vi "LIA_Initialization.vi"(8 "error in (no error)":errorcluster, 10 "Lock-in Parameters":T3[](array[typedef]) {"Value" format="%#_6p"}, 11 "Address":string) -> (0 "error out":errorcluster, 1 "Selected Device":string, 2 "DAQ ModHandle Out":T1 {"ModHandle" format="0x%08x"; "Conn" format="0x%08x"}, 3 "Handle Out":T2 {"Handle" format="0x%08x"; "Conn" format="0x%08x"})   [LabVIEW 2016, in "ZI LIA.lvlib"]
uses:
  ZI LIA.lvlib
  Ctl_SetParameter(Value).ctl
  <instrlib>/Zurich Instruments LabOne/Public/ziTypeHandle.ctl
  <instrlib>/Zurich Instruments LabOne/Public/Modules/ziTypeModHandle.ctl
  <instrlib>/Zurich Instruments LabOne/Public/Modules/ziTypeModEnum.ctl
  <instrlib>/Zurich Instruments LabOne/Public/Configure/ziSetValueDoubleArray.vi
  <instrlib>/Zurich Instruments LabOne/Zurich Instruments LabOne.lvlib
  General.lvlib
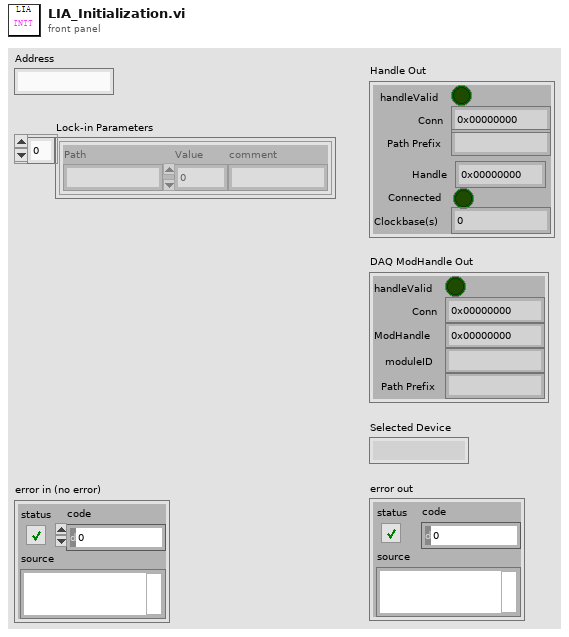
[diagram p1: front panel]
types:
  T1 = typedef "Zurich Instruments LabOne.lvlib/ziTypeModHandle.ctl" = cluster{"handleValid":bool, "Conn":u64, "ModHandle":u64, "moduleID":string, "Path Prefix":string}
  T2 = typedef "Zurich Instruments LabOne.lvlib/ziTypeHandle.ctl" = cluster{"handleValid":bool, "Conn":u64, "Path Prefix":string, "Handle":u64, "Connected":bool, "Clockbase(s)":dbl}
  T3 = typedef "General.lvlib/Ctl_SetParameter(Value).ctl" = cluster{"Path":string, "Value":dbl, "comment":string}
  T4 = typedef "Zurich Instruments LabOne.lvlib/ziTypeModEnum.ctl" = u16
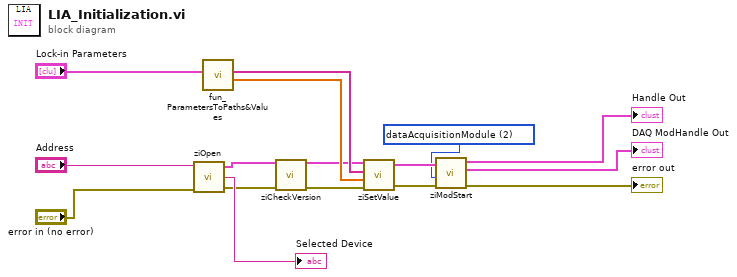
[diagram p0: block diagram]
diagram:
  w11 = T4 2 items=["sweep", "scopeModule", "dataAcquisitionModule", "pidAdvisor", "awgModule", "impedanceModule", "multiDeviceSyncModule", "zoomFFT", "trigger", "deviceSettings", "record"] ("module Id")
  n1 = call <instrlib>:"ziOpen.vi"("Error In"="error in (no error)", "Address"="Address") -> ("Error Out"=w9:errorcluster, "Selected Device"=→"Selected Device":string, "HandleOut"=w6:T2)  [unwired: 2 out]
  n2 = call "fun_ParametersToPaths&Values.vi"("Parameters"="Lock-in Parameters") -> ("Values"=w14:dbl[], "Paths"=w13:string[])  [unwired: 9 in]
  n3 = call <instrlib>:"ziCheckVersion.vi"("Handle In"=w6, "Error In"=w9) -> ("Handle Out"=w7:T2, "Error Out"=w8:errorcluster)  [unwired: 11 in, 1 out]
  n4 = call-poly <instrlib>:"ziSetValue.vi"("Error In"=w8, "Values"=w14, "Paths"=w13, "Handle In"=w7) -> ("Error Out"=w16:errorcluster, "Handle Out"=w15:T2)  [unwired: 1 in]
  n5 = call <instrlib>:"ziModStart.vi"("Error In"=w16, "module Id"=w11, "Handle In"=w15) -> ("Error Out"=→"error out":errorcluster, "ModHandle Out"=→"DAQ ModHandle Out":T1, "Handle Out"=→"Handle Out":T2)  [unwired: 6 in]
